vi "ErrorCase.vi"   [LabVIEW 2014, in "Raspberry Pi Compatible Compiler for LabVIEW.lvlib" / "CaseStructure.lvclass"]
uses:
  CaseStructure.lvclass
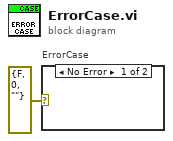
[diagram p0: block diagram]
diagram:
  n1 = case "ErrorCase" shown="No Error" errorcluster {"status"=FALSE, "code"=0, "source"=""} ("error constant") {
    frame No Error {
    }
    frame Error {
    }
  }
